vi "TCPIPInitial.vi"(11 "Enum":enum16{"initial", "Read", "release"}(ring)=enum."release") -> (0 "SN_ReplyRef":refnum<vi>[](array[refnum]), 1 "Connect":refnum<vi>[](array[refnum]), 2 "Sn_cmdQ":refnum<queue>[](array[refnum]), 3 "SN_Reply":refnum<queue>[](array[refnum]))   [LabVIEW 2019]
panel:
  in  "Boolean 5":bool
  in  "Boolean 4":bool
  in  "Boolean 3":bool
  in  "Boolean 2":bool
  in  "Boolean":bool
  in  "String 5":string
  in  "String 4":string
  in  "String 3":string
  in  "String 2":string
  in  "String":string
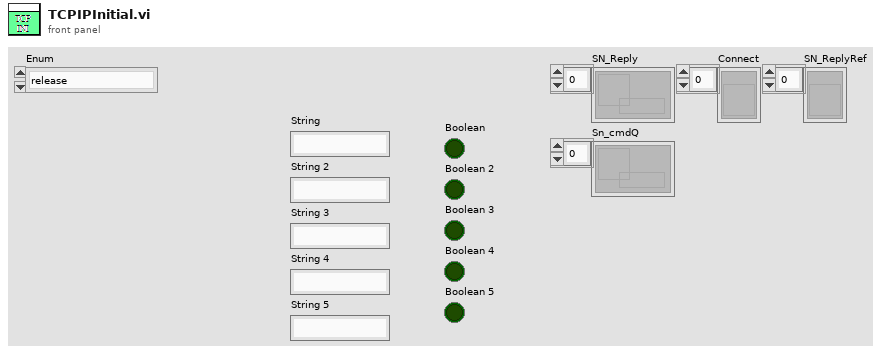
[diagram p1: front panel]
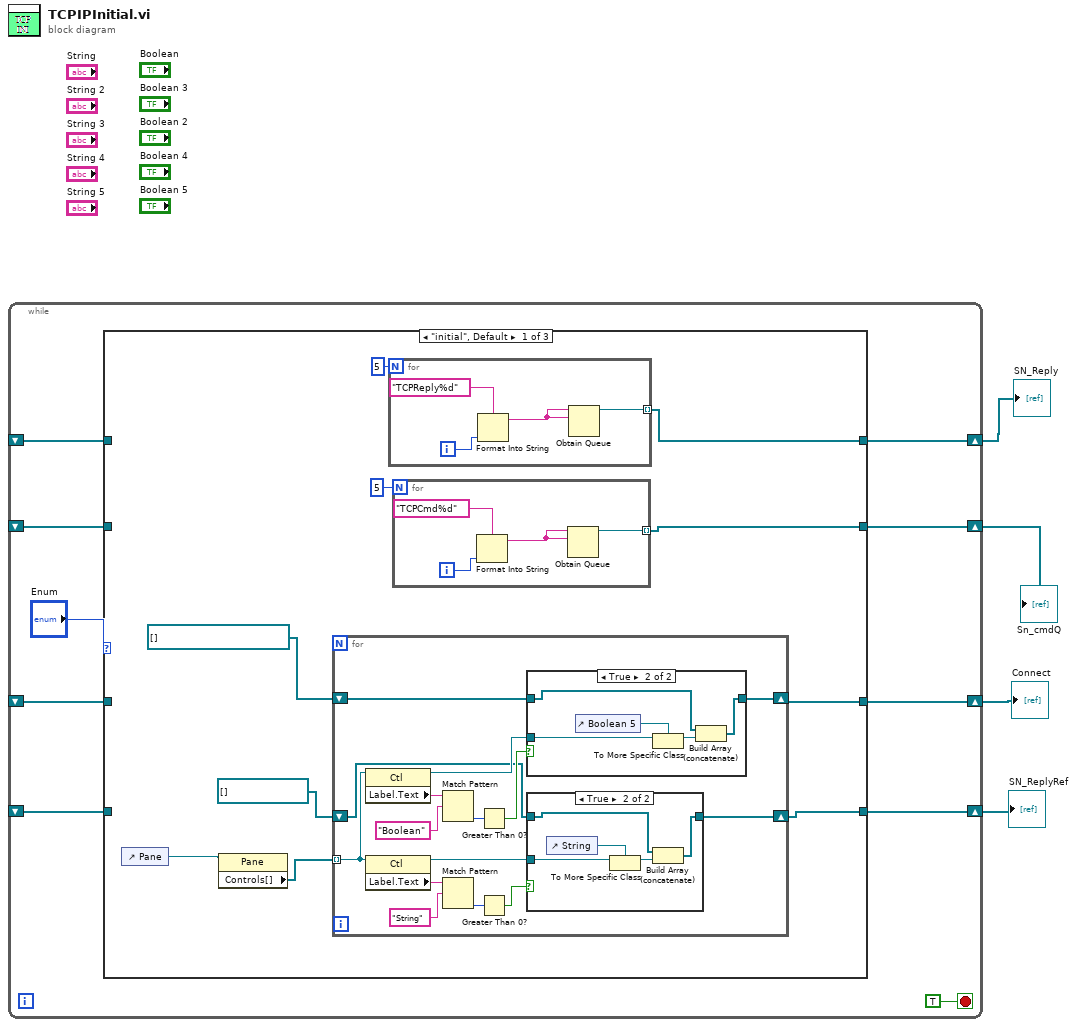
[diagram p0: block diagram]
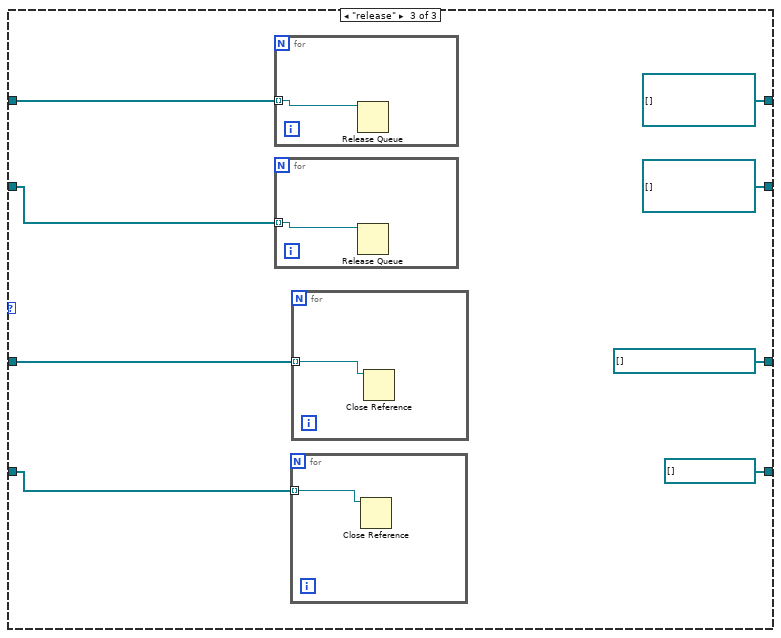
[diagram p5: hidden frame]
diagram:
  n1 = while {
    shift-right: [w12] -> w1
    shift-left: _ -> [w5]
    shift-right: [w11] -> w2
    shift-left: _ -> [w6]
    shift-right: [w13] -> w3
    shift-left: _ -> [w7]
    shift-right: [w14] -> w4
    shift-left: _ -> [w8]
    stop <- TRUE stop-if-true
    n2 = case shown="\"initial\", Default" "Enum" {
      tunnel: [w20 w60 refnum<vi>[] []] -> w14
      tunnel: [w19 w61 refnum<vi>[] []] -> w13
      tunnel: [w16 w63 refnum<queue>[] []] -> w12
      tunnel: [w15 w62 refnum<queue>[] []] -> w11
      tunnel: w8 -> [_ w60 w68]
      tunnel: w7 -> [_ w61 w69]
      tunnel: w6 -> [_ w62 w70]
      tunnel: w5 -> [_ w63 w71]
      frame "initial", Default {
        n3 = control-ref of="Pane"() -> (w24:refnum<vi>)
        n4 = property class="Pane"(reference=w24) -> ("Controls[]"=w23:refnum<vi>[])  [unwired: 1 in, 2 out]
        n5 = for {
          tunnel: w23 -> [w38] mode=indexing
          shift-right: [w42] -> w19
          shift-left: refnum<vi>[] [] -> [w41]
          shift-right: [w33] -> w20
          shift-left: refnum<vi>[] [] -> [w34]
          n6 = property class="Ctl"(reference=w38) -> (reference out=w43:refnum<vi>, "Label.Text"=w47:string)  [unwired: 1 in, 1 out]
          n7 = property class="Ctl"(reference=w38) -> (reference out=w35:refnum<vi>, "Label.Text"=w39:string)  [unwired: 1 in, 1 out]
          n8 = Match Pattern(string=w47, regular expression="Boolean") -> (offset past match=w45:i32)  [unwired: 1 in, 3 out]
          n9 = Match Pattern(string=w39, regular expression="String") -> (offset past match=w37:i32)  [unwired: 1 in, 3 out]
          n10 = Greater Than 0?(x=w45) -> (x > 0?=w44:bool)
          n11 = Greater Than 0?(x=w37) -> (x > 0?=w36:bool)
          n12 = case shown="True" w44 {
            tunnel: w43 -> [_ w56]
            tunnel: [w54 w59] -> w42
            tunnel: w41 -> [w54 w58]
            frame False {
            }
            frame True {
              n13 = control-ref of="Boolean 5"() -> (w55:refnum<vi>)
              n14 = To More Specific Class(target class=w55, reference=w56) -> (specific class reference=w57:refnum<vi>)  [unwired: 1 in, 1 out]
              n15 = Build Array (concatenate)(w58, w57) -> (w59:refnum<vi>[])
            }
          }
          n16 = case shown="True" w36 {
            tunnel: w35 -> [_ w51]
            tunnel: [w48 w53] -> w33
            tunnel: w34 -> [w48 w52]
            frame False {
            }
            frame True {
              n17 = control-ref of="String"() -> (w50:refnum<vi>)
              n18 = To More Specific Class(target class=w50, reference=w51) -> (specific class reference=w49:refnum<vi>)  [unwired: 1 in, 1 out]
              n19 = Build Array (concatenate)(w52, w49) -> (w53:refnum<vi>[])
            }
          }
        }
        n20 = for {
          N: 5 -> [_]
          tunnel: [w25] -> w16 mode=indexing
          i -> [w28]
          n21 = Format Into String(format string="TCPReply%d", w28) -> (resulting string=w26:string)  [unwired: 2 in, 1 out]
          n22 = Obtain Queue(name (unnamed)=w26, element data type=w26) -> (queue out=w25:refnum<queue>)  [unwired: 3 in, 2 out]
        }
        n23 = for {
          N: 5 -> [_]
          tunnel: [w29] -> w15 mode=indexing
          i -> [w32]
          n24 = Format Into String(format string="TCPCmd%d", w32) -> (resulting string=w30:string)  [unwired: 2 in, 1 out]
          n25 = Obtain Queue(name (unnamed)=w30, element data type=w30) -> (queue out=w29:refnum<queue>)  [unwired: 3 in, 2 out]
        }
      }
      frame "Read" {
      }
      frame "release" {
        n26 = for {
          tunnel: w71 -> [w75] mode=indexing
          n27 = Release Queue(queue=w75) -> ()  [unwired: 2 in, 3 out]
        }
        n28 = for {
          tunnel: w70 -> [w74] mode=indexing
          n29 = Release Queue(queue=w74) -> ()  [unwired: 2 in, 3 out]
        }
        n30 = for {
          tunnel: w68 -> [w72] mode=indexing
          n31 = Close Reference(reference=w72) -> ()  [unwired: 1 in, 1 out]
        }
        n32 = for {
          tunnel: w69 -> [w73] mode=indexing
          n33 = Close Reference(reference=w73) -> ()  [unwired: 1 in, 1 out]
        }
      }
    }
  }
  "SN_Reply" <- w1
  "Sn_cmdQ" <- w2
  "Connect" <- w3
  "SN_ReplyRef" <- w4
